vi "CheckValidUserEventReference.vi"(8 "error in":errorcluster, 11 "message ref in":refnum<class "CLM_LocalMessage_UserEvent.lvclass">) -> (0 "error out":errorcluster, 2 "valid?":bool, 3 "message ref out":refnum<class "CLM_LocalMessage_UserEvent.lvclass">)   [LabVIEW 2013, in "CLM_LocalMessage_UserEvent.lvclass"]
uses:
  CLM_LocalMessage_UserEvent.lvclass
  CLM_LocalMessage_UserEvent.lvclass/CLM_LocalMessage_UserEvent.ctl
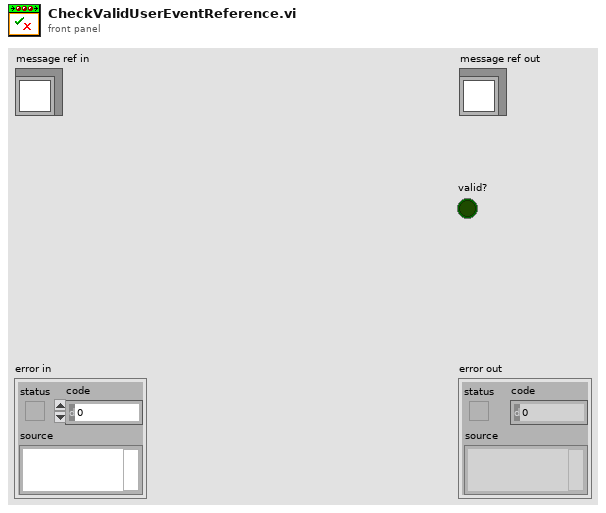
[diagram p1: front panel]
types:
  T1 = typedef "CLM_LocalMessage_UserEvent.lvclass/MessageUserEvent.ctl" = refnum<user-event>
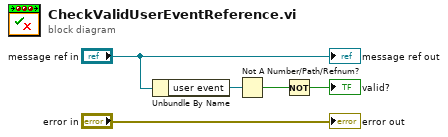
[diagram p0: block diagram]
diagram:
  n1 = Unbundle By Name("message ref in") -> ("user event"=w3:T1)
  n2 = Not A Number/Path/Refnum?(number/path/refnum=w3) -> (NaN/Path/Refnum?=w2:bool)
  n3 = Not(x=w2) -> (.not. x?=→"valid?":bool)
  "error out" <- "error in"
  "message ref out" <- "message ref in"
